vi "CreateMissingItemParentItemInList.vi"(8 "error in (no error)":errorcluster, 11 "CDependencyList in":refnum<class "CDependencyList.lvclass">) -> (0 "error out":errorcluster, 3 "CDependencyList out":refnum<class "CDependencyList.lvclass">)   [LabVIEW 2020, in "DependencyInspection.lvlib" / "CDependencyList.lvclass"]
uses:
  CDependencyList/CDependencyList.lvclass
  LabVIEWObjectFactory/LabVIEWObjectFactory.lvlib
  LabVIEWObjectInterfaces/ILabVIEWItem/ILabVIEWItem.lvclass
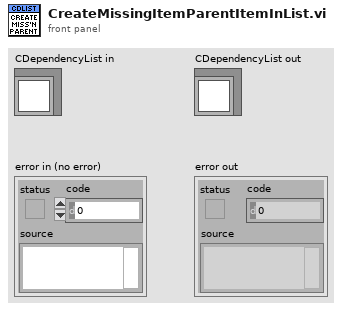
[diagram p1: front panel]
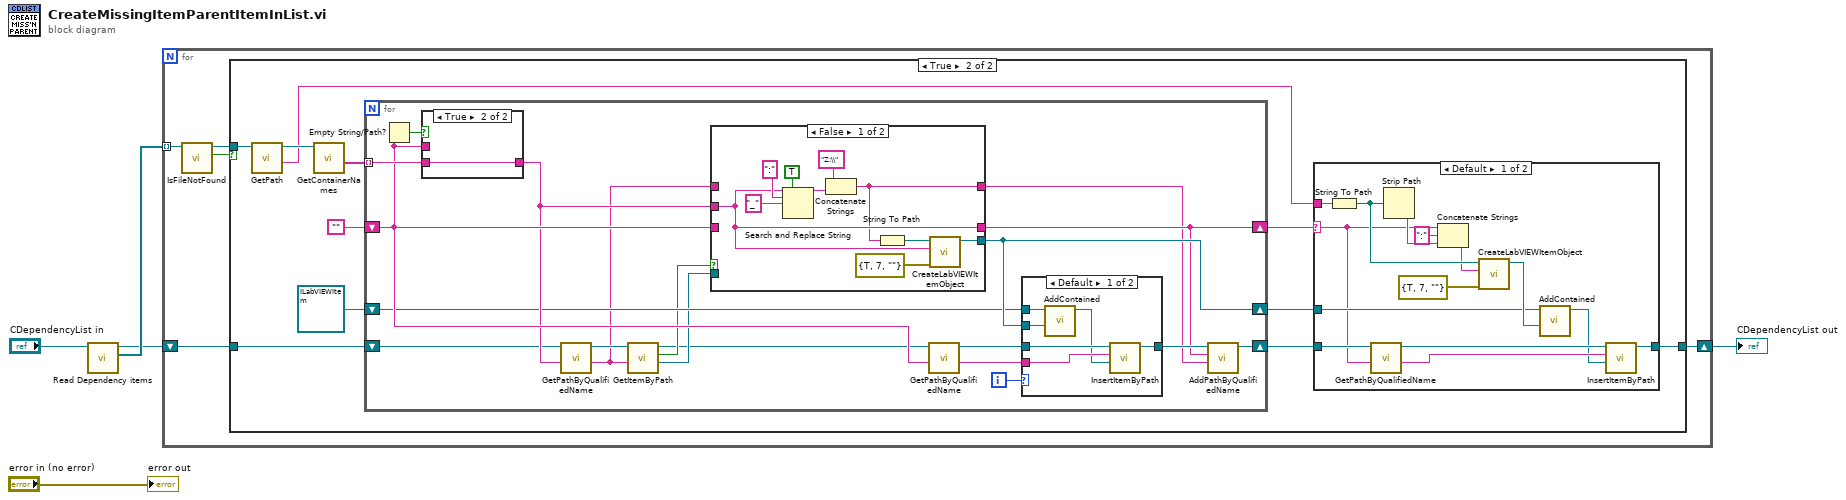
[diagram p0: block diagram]
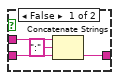
[diagram p3: hidden frame]
diagram:
  n1 = call-dynamic "Read Dependency items.vi"("CDependencyList in"="CDependencyList in") -> ("Dependency items"=w3:refnum<class "ILabVIEWItem.lvclass">[], "CDependencyList out"=w2:refnum<class "CDependencyList.lvclass">)  [unwired: 9 in]
  n2 = for {
    shift-right: [w7] -> w1
    shift-left: w2 -> [w8]
    tunnel: w3 -> [w6] mode=indexing
    n3 = call-dynamic "IsFileNotFound.vi"("ILabVIEWItem in"=w6) -> ("Is file not found?"=w10:bool, "ILabVIEWItem out"=w9:refnum<class "ILabVIEWItem.lvclass">)  [unwired: 8 in, 1 out]
    n4 = case shown="True" w10 {
      tunnel: w9 -> [_ w19]
      tunnel: w8 -> [w11 w21]
      tunnel: [w11 w14] -> w7
      frame False {
      }
      frame True {
        n5 = call-dynamic "GetPath.vi"("ILabVIEWItem in"=w19) -> ("Path"=w16:string, "ILabVIEWItem out"=w18:refnum<class "ILabVIEWItem.lvclass">)  [unwired: 8 in, 1 out]
        n6 = call-dynamic "GetContainerNames.vi"("ILabVIEWItem in"=w18) -> ("Container name[]"=w17:string[])  [unwired: 8 in, 2 out]
        n7 = for {
          tunnel: w17 -> [w41] mode=indexing
          shift-right: [w27] -> w12
          shift-left: "" -> [w37]
          shift-right: [w28] -> w15
          shift-left: w21 -> [w25]
          shift-right: [w38] -> w13
          shift-left: refnum<class "ILabVIEWItem.lvclass"> refnum ("ILabVIEWItem") -> [w34]
          i -> [w39]
          n8 = Empty String/Path?(string/path=w37) -> (empty?=w40:bool)
          n9 = case shown="True" w40 {
            tunnel: w41 -> [w44 w46]
            tunnel: [w42 w46] -> w35
            tunnel: w37 -> [w45 _]
            frame False {
              n10 = Concatenate Strings(w45, ":" ("string"), w44) -> (w42:string)
            }
            frame True {
            }
          }
          n11 = call-dynamic "GetPathByQualifiedName.vi"("Qualified name"=w35, "CDependencyList in"=w25) -> ("Path"=w32:string, "CDependencyList out"=w33:refnum<class "CDependencyList.lvclass">)  [unwired: 6 in, 2 out]
          n12 = call-dynamic "GetItemByPath.vi"("Path"=w32, "CDependencyList in"=w33) -> ("ILabVIEWItem"=w30:refnum<class "ILabVIEWItem.lvclass">, "key found?"=w31:bool, "CDependencyList out"=w24:refnum<class "CDependencyList.lvclass">)  [unwired: 6 in, 1 out]
          n13 = case shown="False" w31 {
            tunnel: w30 -> [_ w59]
            tunnel: [w55 w59] -> w38
            tunnel: w37 -> [_ _]
            tunnel: w35 -> [w48 w58]
            tunnel: [w48 w58] -> w27
            tunnel: [w47 w57] -> w26
            tunnel: w32 -> [_ w57]
            frame False {
              n14 = Search and Replace String(replace all?=TRUE ("replace all? (F)"), input string=w48, search string=":", replace string="_" ("replace string (\"\")")) -> (result string=w54:string)  [unwired: 4 in, 3 out]
              n15 = Concatenate Strings("Z:\\" ("string"), w54) -> (w47:string)
              n16 = String To Path(string=w47) -> (path=w49:path)
              n17 = call "CreateLabVIEWItemObject.vi"("error in (no error)"=errorcluster {"status"=TRUE, "code"=7, "source"=""}, "delimited name"=w48, "SubVI path"=w49) -> ("ILabVIEWItem"=w55:refnum<class "ILabVIEWItem.lvclass">)  [unwired: 7 in, 1 out]
            }
            frame True {
            }
          }
          n18 = call-dynamic "GetPathByQualifiedName.vi"("Qualified name"=w37, "CDependencyList in"=w24) -> ("Path"=w36:string, "CDependencyList out"=w23:refnum<class "CDependencyList.lvclass">)  [unwired: 6 in, 2 out]
          n19 = case shown="Default" w39 {
            tunnel: w38 -> [w64 _]
            tunnel: w23 -> [w63 w66]
            tunnel: [w62 w66] -> w29
            tunnel: w34 -> [w65 _]
            tunnel: w36 -> [w61 _]
            frame Default {
              n20 = call-dynamic "AddContained.vi"("Item to contain"=w64, "ILabVIEWItem in"=w65) -> ("ILabVIEWItem out"=w60:refnum<class "ILabVIEWItem.lvclass">)  [unwired: 7 in, 2 out]
              n21 = call-dynamic "InsertItemByPath.vi"("ILabVIEWItem in"=w60, "Path"=w61, "CDependencyList in"=w63) -> ("CDependencyList out"=w62:refnum<class "CDependencyList.lvclass">)  [unwired: 7 in, 1 out]
            }
            frame 0 {
            }
          }
          n22 = call-dynamic "AddPathByQualifiedName.vi"("Path"=w26, "Qualified name"=w27, "CDependencyList in"=w29) -> ("CDependencyList out"=w28:refnum<class "CDependencyList.lvclass">)  [unwired: 7 in, 1 out]
        }
        n23 = case shown="Default" w12 {
          selector: w12 -> [w71 _]
          tunnel: w16 -> [w79 _]
          tunnel: w15 -> [w72 w81]
          tunnel: [w67 w81] -> w14
          tunnel: w13 -> [w73 _]
          frame Default {
            n24 = String To Path(string=w79) -> (path=w76:path)
            n25 = call-dynamic "GetPathByQualifiedName.vi"("Qualified name"=w71, "CDependencyList in"=w72) -> ("Path"=w69:string, "CDependencyList out"=w70:refnum<class "CDependencyList.lvclass">)  [unwired: 6 in, 2 out]
            n26 = Strip Path(path=w76) -> (name=w77:string)  [unwired: 1 out]
            n27 = Concatenate Strings(w71, ":" ("string"), w77) -> (w75:string)
            n28 = call "CreateLabVIEWItemObject.vi"("error in (no error)"=errorcluster {"status"=TRUE, "code"=7, "source"=""}, "delimited name"=w75, "SubVI path"=w76) -> ("ILabVIEWItem"=w74:refnum<class "ILabVIEWItem.lvclass">)  [unwired: 7 in, 1 out]
            n29 = call-dynamic "AddContained.vi"("Item to contain"=w74, "ILabVIEWItem in"=w73) -> ("ILabVIEWItem out"=w68:refnum<class "ILabVIEWItem.lvclass">)  [unwired: 7 in, 2 out]
            n30 = call-dynamic "InsertItemByPath.vi"("ILabVIEWItem in"=w68, "Path"=w69, "CDependencyList in"=w70) -> ("CDependencyList out"=w67:refnum<class "CDependencyList.lvclass">)  [unwired: 7 in, 1 out]
          }
          frame "" {
          }
        }
      }
    }
  }
  "CDependencyList out" <- w1
  "error out" <- "error in (no error)"
